vi "Get Photosets.vi"(11 "Flickr Ref":refnum<k24>) -> (1 "Names":string[](array[string]), 2 "ids":string[](array[string]), 3 "Flickr Ref out":refnum<k24>)   [LabVIEW 2010]
uses:
  C:/Users/telsey/Desktop/Personal Projects/Photobooth/Flickr API/FlickrNet-3.5.0/FlickrNet.dll
  FlickrNet.dll
  <vilib>/xml/Close Reference(Node).vi
  <vilib>/xml/NI_XML.lvlib
  Program Files (x86)/National Instruments/LabVIEW 2010/resource/objmgr/DOMUserDefRef.rc
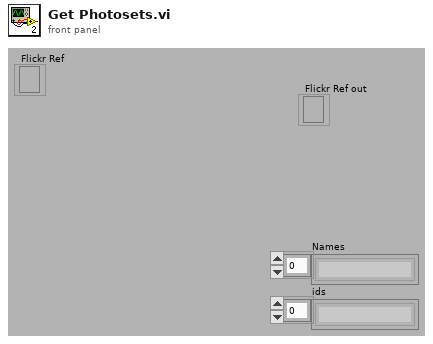
[diagram p1: front panel]
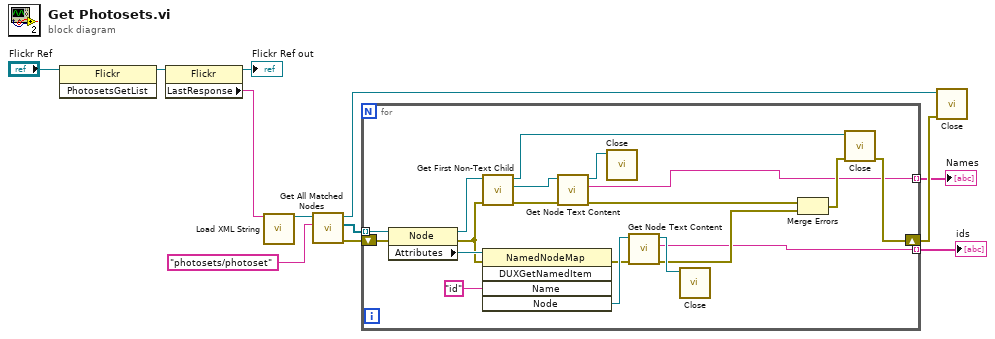
[diagram p0: block diagram]
diagram:
  n1 = invoke class="Flickr" method="PhotosetsGetList"(reference="Flickr Ref") -> (reference out=w4:refnum<k24>)  [unwired: 2 in, 2 out]
  n2 = property class="Flickr"(reference=w4) -> (reference out=→"Flickr Ref out":refnum<k24>, "LastResponse"=w2:string)  [unwired: 1 in, 1 out]
  n3 = call <vilib>:"Load XML String.vi"("XML string"=w2) -> ("DOM document out"=w12:refnum<k20>)  [unwired: 1 in, 13 out]
  n4 = call <vilib>:"Get All Matched Nodes.vi"("XPath expression"="photosets/photoset", "node in"=w12) -> ("error out"=w8:errorcluster, "node result array"=w10:refnum<k20>[], "node out"=w11:refnum<k20>)  [unwired: 1 in, 6 out]
  n5 = for {
    tunnel: w10 -> [w28] mode=indexing
    tunnel: [w14] -> w6 mode=indexing
    shift-right: [w15] -> w7
    shift-left: w8 -> [w22]
    tunnel: [w13] -> w5 mode=indexing
    n6 = property class="Node"(reference=w28, error in=w22) -> (reference out=w26:refnum<k20>, error out=w21:errorcluster, "Attributes"=w31:refnum<k20>)
    n7 = call <vilib>:"Get First Non-Text Child.vi"("error in (no error)"=w21, "node in"=w26) -> ("error out"=w19:errorcluster, "child node"=w25:refnum<k20>, "node out"=w27:refnum<k20>)  [unwired: 6 in, 1 out]
    n8 = invoke class="NamedNodeMap" method="DUXGetNamedItem"(reference=w31, error in=w21, "Name"="id") -> (error out=w20:errorcluster, "Node"=w29:refnum<k20>)  [unwired: 2 in, 3 out]
    n9 = call <vilib>:"Get Node Text Content.vi"("error in (no error)"=w19, "node in"=w25) -> ("error out"=w18:errorcluster, "node text"=w14:string, "node out"=w24:refnum<k20>)  [unwired: 7 in]
    n10 = call-poly <vilib>:"Close.vi"("node"=w24) -> ()  [unwired: 1 in, 8 out]
    n11 = call <vilib>:"Get Node Text Content.vi"("error in (no error)"=w20, "node in"=w29) -> ("error out"=w17:errorcluster, "node text"=w13:string, "node out"=w23:refnum<k20>)  [unwired: 7 in]
    n12 = call-poly <vilib>:"Close.vi"("node"=w23) -> ()  [unwired: 1 in, 8 out]
    n13 = Merge Errors(w18, w17) -> (w16:errorcluster)
    n14 = call-poly <vilib>:"Close.vi"("error in (no error)"=w16, "node"=w27) -> ("error out"=w15:errorcluster)  [unwired: 7 out]
  }
  "Names" <- w6
  "ids" <- w5
  n15 = call-poly <vilib>:"Close.vi"("error in (no error)"=w7, "node"=w11) -> ()  [unwired: 7 in, 1 out]
